vi "Add ECO For DLL-SD.vi"(1 "x":u32) -> (0 "x + ECO4DLL":u32)   [LabVIEW 2018, in "CCD_camera.lvclass"]
doc: "Adds the <B>ECO For DLL</B> to the input value."
uses:
  CCD_camera.lvclass
  Error Code Offset globalSD.vi
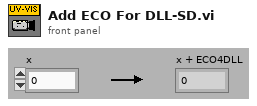
[diagram p1: front panel]
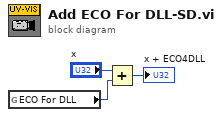
[diagram p0: block diagram]
diagram:
  n1 = global read "Error Code Offset globalSD.vi" "ECO For DLL"() -> (w1:u32)
  n2 = Add(x="x", y=w1) -> (x+y=→"x + ECO4DLL":u32)
